vi "Write Color.vi"(8 "error in (no error)":errorcluster, 10 "Color in":u32(colorbox), 11 "Shapeable in":refnum<class "Shapeable.lvclass">) -> (0 "error out":errorcluster, 3 "Shapeable out":refnum<class "Shapeable.lvclass">)   [LabVIEW 2022 SP3, in "Shapeable.lvclass"]
uses:
  Shapeable.lvclass
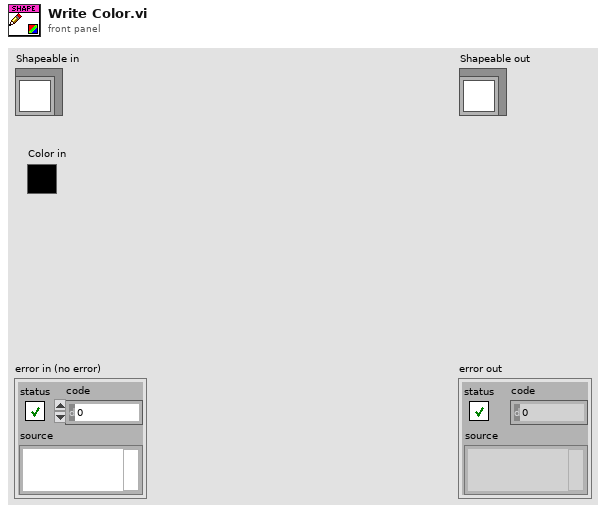
[diagram p1: front panel]
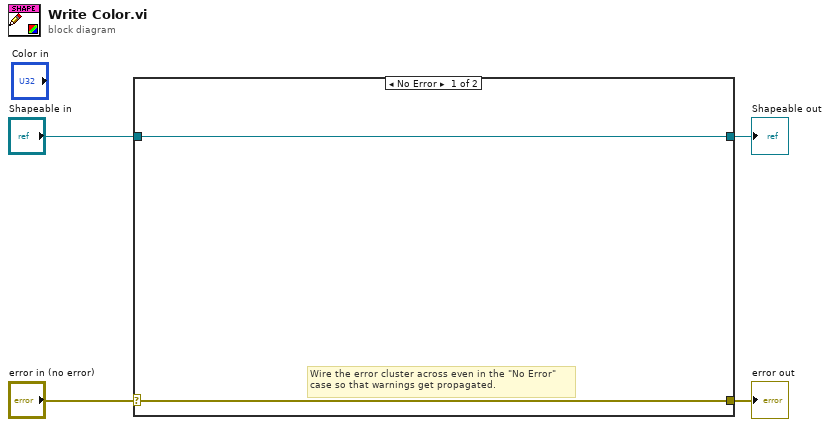
[diagram p0: block diagram]
diagram:
  n1 = case shown="No Error" "error in (no error)" {
    selector: "error in (no error)" -> [w5 w8]
    tunnel: [w5 w8] -> w3
    tunnel: [w6 w7] -> w1
    tunnel: "Shapeable in" -> [w6 w7]
    frame No Error {
      # "Wire the error cluster across even in the \"No Error\"\ncase so that warnings get propagated."
    }
    frame Error {
    }
  }
  "error out" <- w3
  "Shapeable out" <- w1
